vi "Findh.vi"(0 "Full h(r,t)":bool, 1 "Trans Geometry":cluster{"Radius (cm)":dbl, "a (cm)":dbl}={"Radius (cm)"=4.8, "a (cm)"=1.0} {"a (cm)" format="%.2f"; "Radius (cm)" format="%.2f"}, 4 "Variables in":T1={"Number of rings"=1, "sound spd (cm/s)"=150000, "z span (cm)"=4.0, "z steps"=20, "y span (cm)"=50.0, "y steps"=0, "time step (s)"=1e-08, "z"=0.0, "y"=0.0, "ref delay"=0.0, "freq (MHz)"=4.71, "cycles"=300} {"freq (MHz)" format="%.2f"; "z span (cm)" format="%.2f"; "y" format="%.2f"; "ref delay" format="%.2f"; "y span (cm)" format="%.2f"; "z" format="%.2f"; "time step (s)" format="%.2e"}) -> (5 "h(r,t)":dbl[](graph), 6 "beta(t)/2":dbl[](array[numeric]) format="%.2f", 7 "delay pts":i32)   [LabVIEW 2022 SP3]
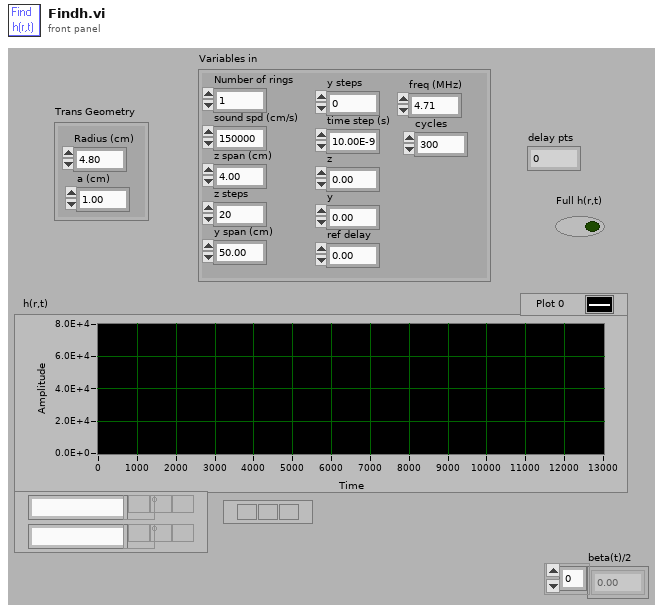
[diagram p1: front panel]
types:
  T1 = cluster{"Number of rings":i32, "sound spd (cm/s)":i32, "z span (cm)":dbl, "z steps":i32, "y span (cm)":dbl, "y steps":i32, "time step (s)":sgl, "z":dbl, "y":dbl, "ref delay":dbl, "freq (MHz)":dbl, "cycles":i32}
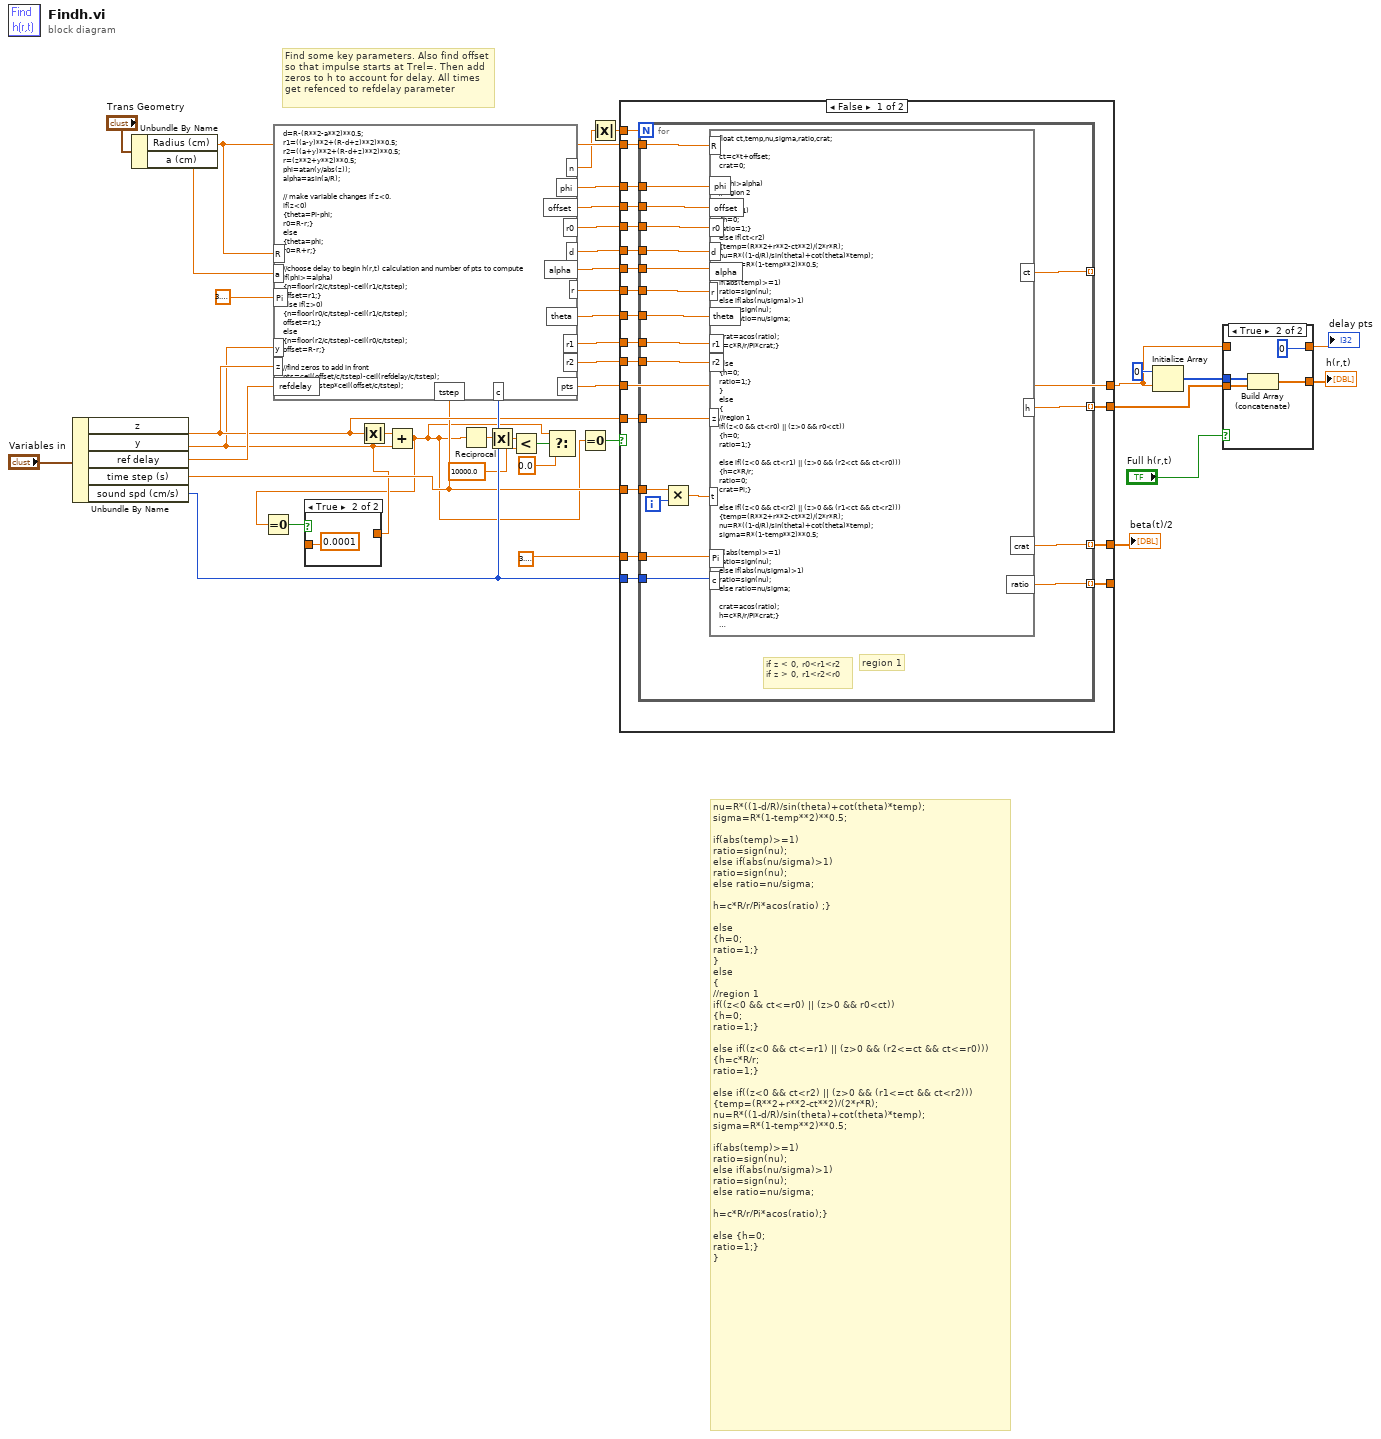
[diagram p0: block diagram]
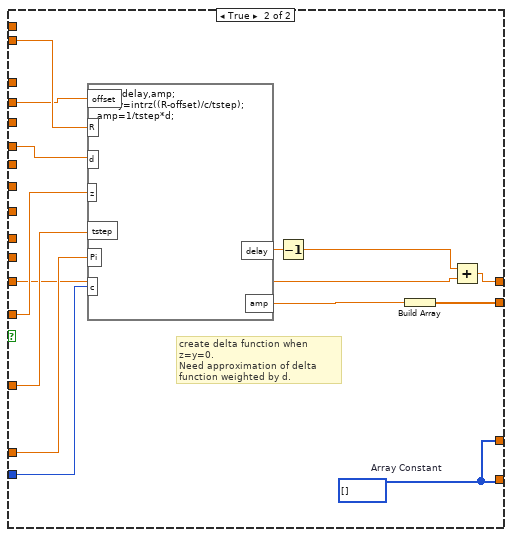
[diagram p4: hidden frame]
diagram:
  # "nu=R*((1-d/R)/sin(theta)+cot(theta)*temp);\nsigma=R*(1-temp**2)**0.5;\n\nif(abs(temp)>=1)\nratio=sign(nu);\nelse if(abs(nu/sigma)>1)\nratio=sign(nu);\nelse ratio=nu/sigma;\n\nh=c*R/r/Pi*acos(ratio) ;}\n\nelse \n{h=0;\nratio=1;}\n}\nelse\n{\n//region 1\nif((z<0 && ct<=r0) || (z>0 && r0<ct))\n{h=0;\nratio=1;}\n\nelse if((z<0 && ct<=r1) || (z>0 && (r2<=ct && ct<=r0)))\n{h=c*R/r;\nratio=1;}\n\nelse if((z<0 && ct<r2) || (z>0 && (r1<=ct && ct<r2)))\n{temp=(R**2+r**2-ct**2)/(2*r*R);\nnu=R*((1-d/R)/sin(theta)+cot(theta)*temp);\nsigma=R*(1-temp**2)**0.5;\n\nif(abs(temp)>=1)\nratio=sign(nu);\nelse if(abs(nu/sigma)>1)\nratio=sign(nu);\nelse ratio=nu/sigma;\n\nh=c*R/r/Pi*acos(ratio);}\n\nelse {h=0;\nratio=1;}\n}"
  # "Find some key parameters. Also find offset so that impulse starts at Trel=. Then add zeros to h to account for delay. All times get refenced to refdelay parameter"
  n1 = Unbundle By Name("Variables in") -> ("z"=w26:dbl, "y"=w3:dbl, "ref delay"=w28:dbl, "time step (s)"=w5:sgl, "sound spd (cm/s)"=w27:i32)
  n2 = Unbundle By Name("Trans Geometry") -> ("Radius (cm)"=w38:dbl, "a (cm)"=w37:dbl)
  n3 = formula code="d=R-(R**2-a**2)**0.5;\nr1=((a-y)**2+(R-d+z)**2)**0.5;\nr2=((a+y)**2+(R-d+z)**2)**0.5;\nr=(z**2+y**2)**0.5;\nphi=atan(y/abs(z));\nalpha=asin(a/R);\n\n// make variable changes if z<0. \nif(z<0) \n{theta=Pi-phi;\nr0=R-r;}\nelse \n{theta=phi;\nr0=R+r;}\n\n//choose delay to begin h(r,t) calculation and number of pts to compute\nif(phi>=alpha)\n{n=floor(r2/c/tstep)-ceil(r1/c/tstep);\noffset=r1;}\nelse if(z>0)\n{n=floor(r0/c/tstep)-ceil(r1/c/tstep);\noffset=r1;}\nelse\n{n=floor(r2/c/tstep)-ceil(r0/c/tstep);\noffset=R-r;}\n\n//find zeros to add in front\npts=ceil(offset/c/tstep)-ceil(refdelay/c/tstep);\noffset=c*tstep*ceil(offset/c/tstep);"("a"=w37, "y"=w3, "R"=w38, "z"=w26, "tstep"=w5, "refdelay"=w28, "c"=w27, "Pi"=3.141592653589793) -> ("r1"=w36:dbl, "r2"=w35:dbl, "theta"=w33:dbl, "r"=w34:dbl, "alpha"=w32:dbl, "d"=w31:dbl, "pts"=w19:dbl, "offset"=w8:dbl, "r0"=w23:dbl, "phi"=w24:dbl, "n"=w21:dbl)
  n4 = Absolute Value(x=w26) -> (abs(x)=w25:dbl)
  n5 = Add(x=w25, y=w3) -> (x+y=w1:dbl)
  n6 = Equal To 0?(x=w1) -> (x = 0?=w6:bool)
  n7 = case shown="True" w6 {
    tunnel: [w41 0.0001 ("y")] -> _
    tunnel: w3 -> [w41 _]
    frame False {
    }
    frame True {
    }
  }
  n8 = Reciprocal(x=w1) -> (1/x=w12:dbl)
  n9 = Absolute Value(x=w12) -> (abs(x)=w11:dbl)
  n10 = Less?(x=w11, y=10000.0) -> (x < y?=w10:bool)
  n11 = Select(t=w1, s=w10, f=0.0) -> ()  [unwired: 1 out]
  n12 = Equal To 0?(x=w1) -> (x = 0?=w30:bool)
  n13 = Absolute Value(x=w21) -> (abs(x)=w2:dbl)
  n14 = case shown="False" w30 {
    tunnel: 3.141592653589793 -> [w61 w90]
    tunnel: w38 -> [w60 w95]
    tunnel: w36 -> [w59 _]
    tunnel: w35 -> [w58 _]
    tunnel: w34 -> [w57 _]
    tunnel: w33 -> [w56 _]
    tunnel: w5 -> [w55 w94]
    tunnel: w26 -> [w54 w93]
    tunnel: w32 -> [w53 _]
    tunnel: w31 -> [w52 w92]
    tunnel: w27 -> [w51 w91]
    tunnel: [w50 w83] -> w18
    tunnel: w8 -> [w49 w89]
    tunnel: w24 -> [w48 _]
    tunnel: w23 -> [w47 _]
    tunnel: w2 -> [w46 _]
    tunnel: w19 -> [w45 w87]
    tunnel: [w45 w85] -> w7
    tunnel: [w44 w82] -> _
    tunnel: [w43 w82] -> w13
    frame False {
      n15 = for {
        N: w46 -> [_]
        tunnel: w61 -> [w81]
        tunnel: w51 -> [w80]
        tunnel: w60 -> [w79]
        tunnel: w52 -> [w78]
        tunnel: w59 -> [w77]
        tunnel: w58 -> [w76]
        tunnel: w57 -> [w75]
        tunnel: w56 -> [w74]
        tunnel: w54 -> [w69]
        tunnel: [w73] -> w50 mode=indexing
        tunnel: w55 -> [w70]
        tunnel: w53 -> [w68]
        tunnel: w49 -> [w67]
        tunnel: [w66] -> _ mode=indexing
        tunnel: [w62] -> w44 mode=indexing
        tunnel: w48 -> [w65]
        tunnel: w47 -> [w64]
        tunnel: [w63] -> w43 mode=indexing
        i -> [w72]
        # "if z < 0, r0<r1<r2\nif z > 0, r1<r2<r0"
        # "region 1"
        n16 = Multiply(x=w70, y=w72) -> (x*y=w71:sgl)
        n17 = formula code="float ct,temp,nu,sigma,ratio,crat;\n\nct=c*t+offset;\ncrat=0;\n\nif(phi>alpha)\n//region 2\n{\nif(ct<r1)\n{h=0;\nratio=1;}\nelse if(ct<r2)\n{temp=(R**2+r**2-ct**2)/(2*r*R);\nnu=R*((1-d/R)/sin(theta)+cot(theta)*temp);\nsigma=R*(1-temp**2)**0.5;\n\nif(abs(temp)>=1)\nratio=sign(nu);\nelse if(abs(nu/sigma)>1)\nratio=sign(nu);\nelse ratio=nu/sigma;\n\ncrat=acos(ratio);\nh=c*R/r/Pi*crat;}\n\nelse \n{h=0;\nratio=1;}\n}\nelse\n{\n//region 1\nif((z<0 && ct<r0) || (z>0 && r0<ct))\n{h=0;\nratio=1;}\n\nelse if((z<0 && ct<r1) || (z>0 && (r2<ct && ct<r0)))\n{h=c*R/r;\nratio=0;\ncrat=Pi;}\n\nelse if((z<0 && ct<r2) || (z>0 && (r1<ct && ct<r2)))\n{temp=(R**2+r**2-ct**2)/(2*r*R);\nnu=R*((1-d/R)/sin(theta)+cot(theta)*temp);\nsigma=R*(1-temp**2)**0.5;\n\nif(abs(temp)>=1)\nratio=sign(nu);\nelse if(abs(nu/sigma)>1)\nratio=sign(nu);\nelse ratio=nu/sigma;\n\ncrat=acos(ratio);\nh=c*R/r/Pi*crat;}\n\nelse {h=0;\nratio=1;}\n}"("t"=w71, "r1"=w77, "r2"=w76, "r"=w75, "R"=w79, "d"=w78, "Pi"=w81, "theta"=w74, "c"=w80, "z"=w69, "alpha"=w68, "offset"=w67, "phi"=w65, "r0"=w64) -> ("h"=w73:dbl, "ratio"=w62:dbl, "ct"=w66:dbl, "crat"=w63:dbl)
      }
    }
    frame True {
      w82 = i32[] []  # Array Constant
      # "create delta function when z=y=0.\nNeed approximation of delta function weighted by d."
      n18 = formula code="float delay,amp;\ndelay=intrz((R-offset)/c/tstep);\namp=1/tstep*d;"("z"=w93, "R"=w95, "tstep"=w94, "d"=w92, "c"=w91, "Pi"=w90, "offset"=w89) -> ("delay"=w88:dbl, "amp"=w84:dbl)
      n19 = Decrement(x=w88) -> (x-1=w86:dbl)
      n20 = Build Array(w84) -> (w83:dbl[])
      n21 = Add(x=w86, y=w87) -> (x+y=w85:dbl)
    }
  }
  "beta(t)/2" <- w13
  n22 = Initialize Array(0, w7) -> (w16:i32[])
  n23 = case shown="True" "Full h(r,t)" {
    tunnel: w18 -> [w97 w101]
    tunnel: [w97 w100] -> w17
    tunnel: w16 -> [_ w99]
    tunnel: [w96 0] -> w14
    tunnel: w7 -> [w96 _]
    frame False {
    }
    frame True {
      n24 = Build Array (concatenate)(w99, w101) -> (w100:dbl[])
    }
  }
  "h(r,t)" <- w17
  "delay pts" <- w14
